vi "J1939 Conversion Lookup Table.vi"(6 "command":enum16{"Set All", "Lookup Parameters"}(ring), 8 "error in (no error)":errorcluster {"code" min=0 max=0}, 10 "ID":u32, 11 "scaling information":T1) -> (0 "error out":errorcluster {"code" min=0 max=0}, 1 "Found?":bool, 2 "Parameters":T3)   [LabVIEW 2013, in "J1939.lvlib"]
uses:
  J1939.lvlib
  J1939 Conversion Lookup Table Parameters Cluster.ctl
  API Types/Scaling Initialization.ctl
  CD/CD Conversion Lookup Table Parameters Cluster.ctl
  Frame Conversion/Common Conversions.vi
  Frame Conversion/Convert CAN Arb ID to J1939 ID.vi
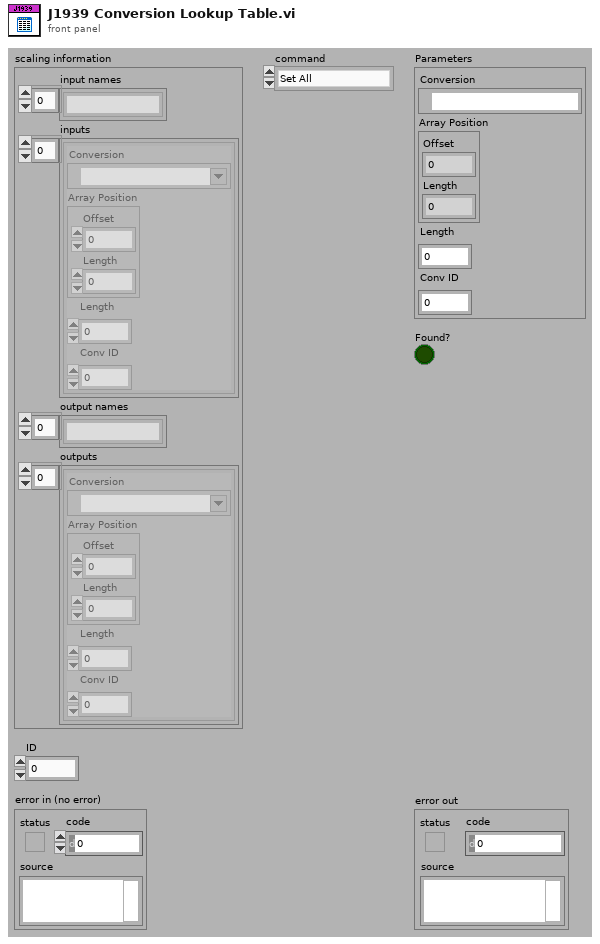
[diagram p1: front panel]
types:
  T1 = typedef "J1939.lvlib/scaling initialization.ctl" = cluster{"input names":string[], "inputs":T2[], "output names":string[], "outputs":T2[]}
  T2 = typedef "J1939.lvlib/CD Conversion Lookup Table Parameters Cluster.ctl" = cluster{"Conversion":refnum<k21>, "Array Position":cluster{"Offset":u32, "Length":u32}, "Length":u32, "Conv ID":u32}
  T3 = typedef "J1939.lvlib/J1939 Conversion Lookup Table Parameters Cluster.ctl" = cluster{"Conversion":refnum<k21>, "Array Position":cluster{"Offset":u32, "Length":u32}, "Length":u32, "Conv ID":u32}
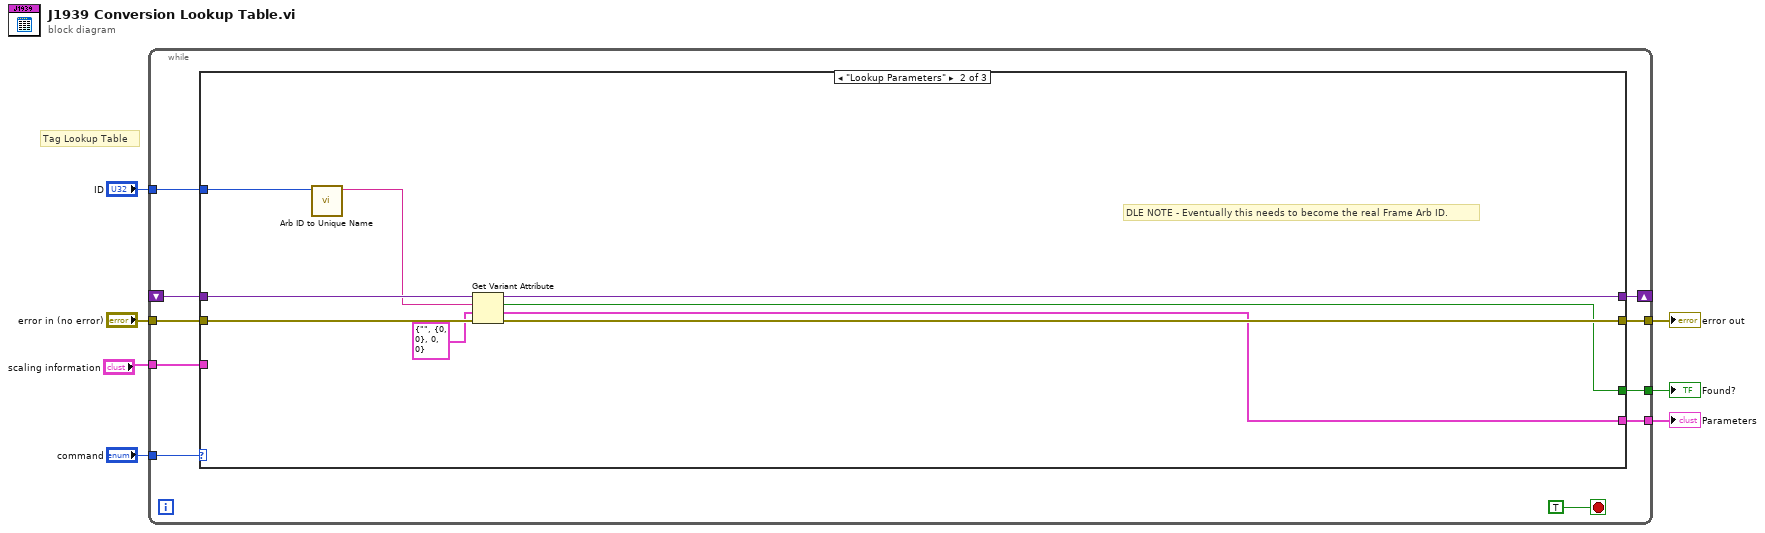
[diagram p0: block diagram]
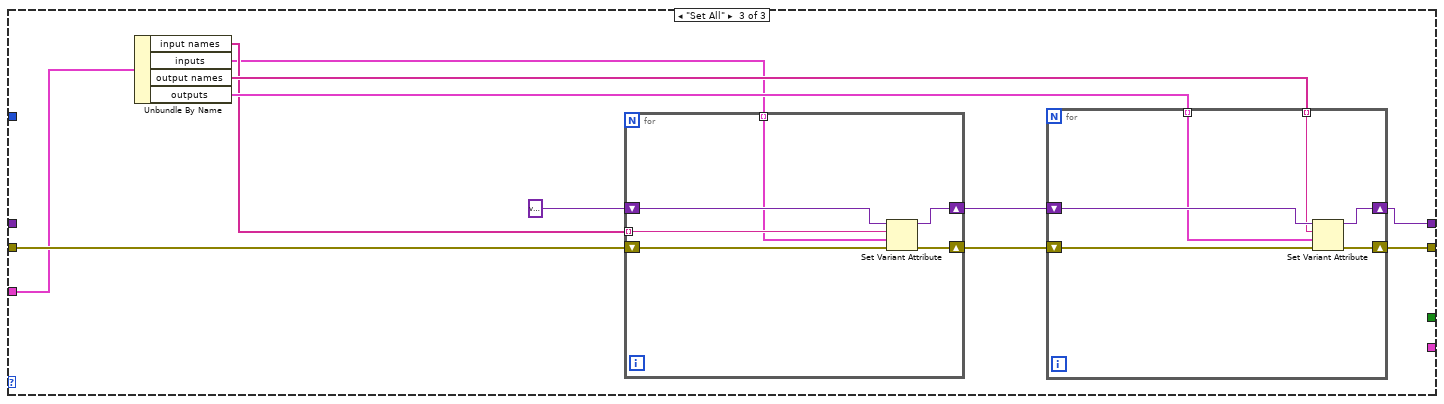
[diagram p3: hidden frame]
diagram:
  # "Tag Lookup Table"
  n1 = while {
    shift-right: [w15] -> _
    shift-left: _ -> [w14]
    tunnel: "command" -> [w16]
    tunnel: "error in (no error)" -> [w13]
    tunnel: [w12] -> w5
    tunnel: "ID" -> [w11]
    tunnel: [w10] -> w3
    tunnel: [w9] -> w2
    tunnel: "scaling information" -> [w8]
    stop <- TRUE stop-if-true
    n2 = case shown="\"Lookup Parameters\"" w16 {
      tunnel: [w18 w25 w33] -> w15
      tunnel: w14 -> [w18 w27 _]
      tunnel: w13 -> [_ w26 w37]
      tunnel: [_ w24 w34] -> w12
      tunnel: w11 -> [_ w20 _]
      tunnel: [_ w23 _] -> w10
      tunnel: [_ w21 _] -> w9
      tunnel: w8 -> [_ _ w32]
      frame Default {
      }
      frame "Lookup Parameters" {
        # "DLE NOTE - Eventually this needs to become the real Frame Arb ID."
        n3 = call "Arb ID to Unique Name.vi"("Arb ID"=w20) -> ("name"=w19:string)  [unwired: 10 in]
        n4 = Get Variant Attribute(Variant=w27, name=w19, default value (empty Variant)=T3 {"Conversion"="", "Array Position"={"Offset"=0, "Length"=0}, "Length"=0, "Conv ID"=0} ("Parameters"), error in=w26) -> (duplicate Variant=w25:variant, found=w21:bool, value=w23:T3, error out=w24:errorcluster)
      }
      frame "Set All" {
        n5 = Unbundle By Name(w32) -> ("input names"=w29:string[], "inputs"=w28:T2[], "output names"=w31:string[], "outputs"=w30:T2[])
        n6 = for {
          shift-right: [w49] -> w36
          shift-left: variant ("variant") -> [w50]
          shift-right: [w47] -> w35
          shift-left: w37 -> [w48]
          tunnel: w29 -> [w46] mode=indexing
          tunnel: w28 -> [w45] mode=indexing
          n7 = Set Variant Attribute(Variant=w50, name=w46, value=w45, error in=w48) -> (Variant out=w49:variant, error out=w47:errorcluster)  [unwired: 1 out]
        }
        n8 = for {
          shift-right: [w43] -> w33
          shift-left: w36 -> [w44]
          shift-right: [w41] -> w34
          shift-left: w35 -> [w42]
          tunnel: w31 -> [w40] mode=indexing
          tunnel: w30 -> [w39] mode=indexing
          n9 = Set Variant Attribute(Variant=w44, name=w40, value=w39, error in=w42) -> (Variant out=w43:variant, error out=w41:errorcluster)  [unwired: 1 out]
        }
      }
    }
  }
  "error out" <- w5
  "Parameters" <- w3
  "Found?" <- w2
